vi "Sets_Union(VAR).vi"(8 "error in (no error)":errorcluster caption="错误输入（无错误）", 10 "输入数组B":variant[](array[variant]), 11 "输入数组A":variant[](array[variant])) -> (0 "error out":errorcluster caption="错误输出", 3 "输出数组C":variant[](array[variant]))   [LabVIEW 2011]
uses:
  Sets_Unique(VAR).vi
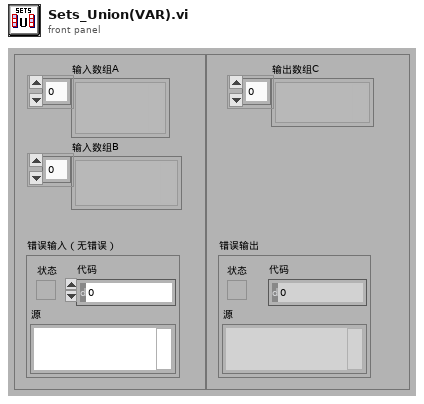
[diagram p1: front panel]
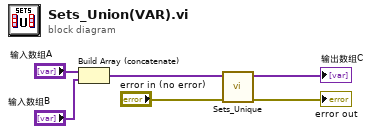
[diagram p0: block diagram]
diagram:
  n1 = Build Array (concatenate)("输入数组A", "输入数组B") -> (w3:variant[])
  n2 = call-poly "Sets_Unique.vi"("error in (no error)"="error in (no error)", "输入数组"=w3) -> ("error out"=→"error out":errorcluster, "输出数组"=→"输出数组C":variant[])  [unwired: 7 in, 1 out]
